vi "eventLogger.vi"() -> ()   [LabVIEW 2017]
panel:
  in  "stop":bool
  in  "enter":bool
  in  "Event text":string
  in  "Rat ID":string
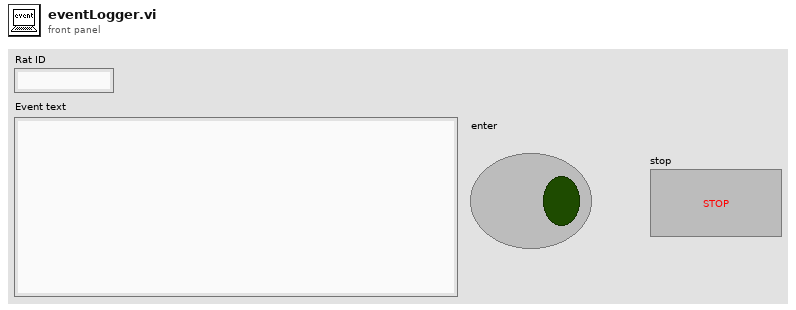
[diagram p1: front panel]
types:
  T1 = enum16{"open", "replace", "create", "open or create", "replace or create", "replace or create with confirmation"}
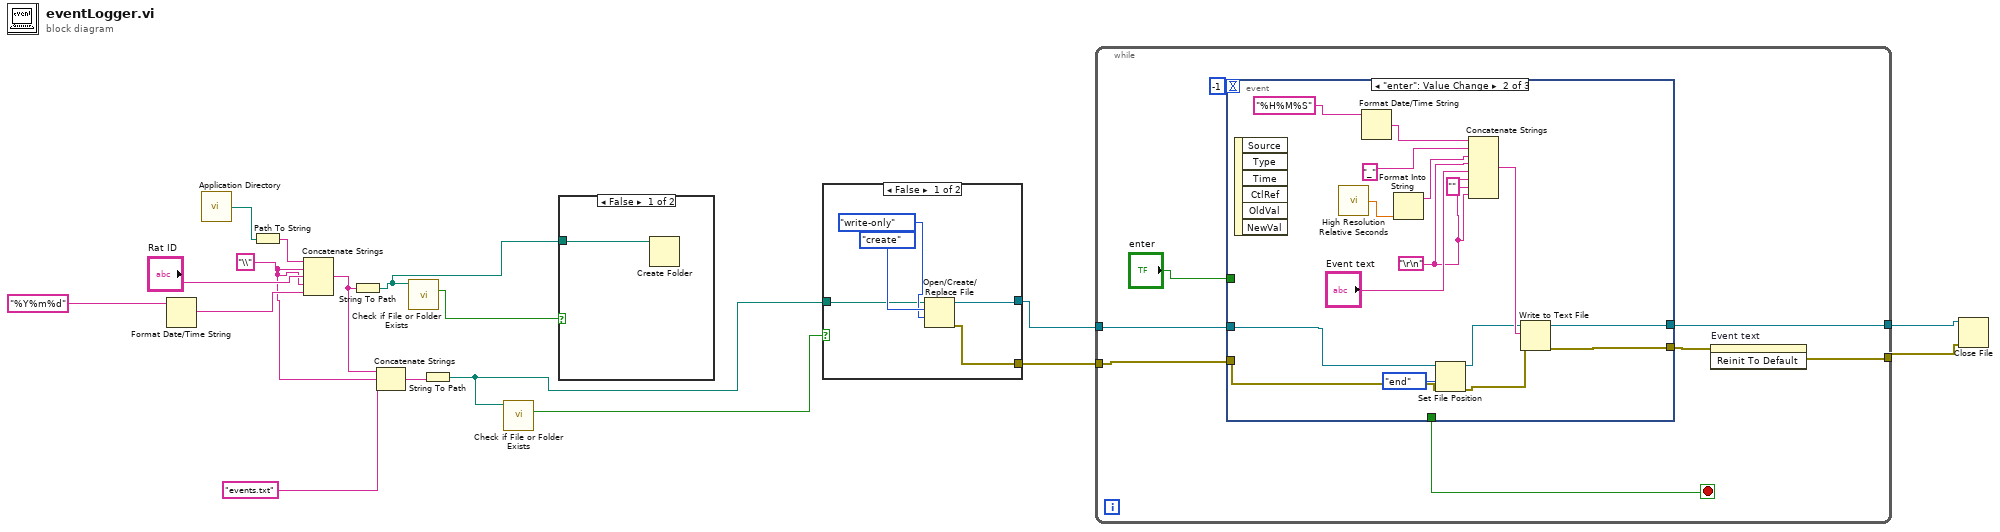
[diagram p0: block diagram]
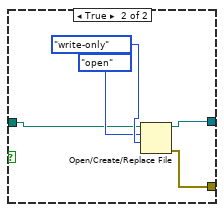
[diagram p2: hidden frame]
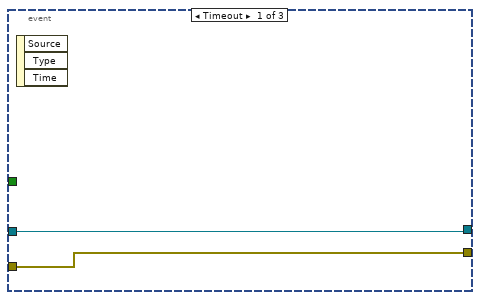
[diagram p4: hidden frame]
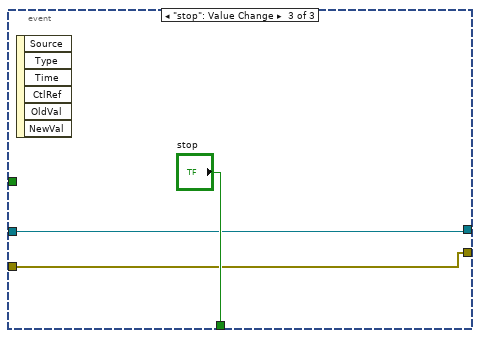
[diagram p5: hidden frame]
diagram:
  w12 = "\\" ("string")
  n1 = Format Date/Time String(time format string (%c)="%Y%m%d" ("time string")) -> (date/time string=w15:string)  [unwired: 2 in]
  n2 = call <vilib>:"Application Directory.vi"() -> ("Application Directory"=w14:path)
  n3 = Path To String(path=w14) -> (string=w17:string)
  n4 = Concatenate Strings(w17, w12, "Rat ID", w12, w15) -> (w11:string)
  n5 = String To Path(string=w11) -> (path=w7:path)
  n6 = Concatenate Strings(w11, w12, "events.txt" ("string")) -> (w9:string)
  n7 = call <vilib>:"Check if File or Folder Exists.vi"("path"=w7) -> ("file or folder exists?"=w8:bool)  [unwired: 8 in, 2 out]
  n8 = String To Path(string=w9) -> (path=w5:path)
  n9 = call <vilib>:"Check if File or Folder Exists.vi"("path"=w5) -> ("file or folder exists?"=w6:bool)  [unwired: 8 in, 2 out]
  n10 = case shown="False" w8 {
    tunnel: w7 -> [w18 _]
    frame False {
      n11 = Create Folder(path (use dialog)=w18) -> ()  [unwired: 2 in, 3 out]
    }
    frame True {
    }
  }
  n12 = case shown="False" w6 {
    tunnel: [w21 w25] -> w4
    tunnel: w5 -> [w20 w26]
    tunnel: [w19 w24] -> w3
    frame False {
      n13 = Open/Create/Replace File(file path (use dialog)=w20, operation (0:open)=T1."create", access (0:read/write)=enum16{"read/write", "read-only", "write-only"}."write-only") -> (refnum out=w21:refnum<file>, error out=w19:errorcluster)  [unwired: 3 in, 1 out]
    }
    frame True {
      n14 = Open/Create/Replace File(file path (use dialog)=w26, operation (0:open)=T1."open", access (0:read/write)=enum16{"read/write", "read-only", "write-only"}."write-only") -> (refnum out=w25:refnum<file>, error out=w24:errorcluster)  [unwired: 3 in, 1 out]
    }
  }
  n15 = while {
    tunnel: w4 -> [w30]
    tunnel: w3 -> [w36]
    tunnel: [w34] -> w2
    tunnel: [w29] -> w1
    stop <- w31 stop-if-true
    n16 = event shown="[1] \"enter\": Value Change" {
      selector: _ -> [_ _ _]
      dyn-events: _ -> [_ _ _]
      timeout: -1 -> [_ _ _]
      tunnel: w36 -> [w38 w49 w55]
      tunnel: [w38 w54 w55] -> w35
      tunnel: "enter" -> [_ _ _]
      tunnel: [_ _ "stop"] -> w31
      tunnel: w30 -> [w37 w46 w56]
      tunnel: [w37 w45 w56] -> w29
      event Timeout {
        n17 = event-data() -> ()  [unwired: 1 in, 3 out]
      }
      event "enter": Value Change {
        w39 = "\r\n"
        n18 = event-data() -> ()  [unwired: 1 in, 6 out]
        n19 = call <vilib>:"High Resolution Relative Seconds.vi"() -> ("relative seconds"=w53:dbl)
        n20 = Format Date/Time String(time format string (%c)="%H%M%S" ("time string")) -> (date/time string=w44:string)  [unwired: 2 in]
        n21 = Format Into String(w53) -> (resulting string=w52:string)  [unwired: 3 in, 1 out]
        n22 = Set File Position(refnum=w46, from (0:start)=enum16{"start", "end", "current"}."end", error in=w49) -> (refnum out=w48:refnum<file>, error out=w50:errorcluster)  [unwired: 1 in]
        n23 = Concatenate Strings(w44, "_" ("string"), w52, w39, "Event text", w39, "" ("string"), w39) -> (w51:string)
        n24 = Write to Text File(file (use dialog)=w48, text=w51, error in=w50) -> (refnum out=w45:refnum<file>, error out=w54:errorcluster)  [unwired: 1 in, 1 out]
      }
      event "stop": Value Change {
        n25 = event-data() -> ()  [unwired: 1 in, 6 out]
      }
    }
    n26 = invoke on="Event text" class="Str" method="Reinit To Default"(error in=w35) -> (error out=w34:errorcluster)  [unwired: 2 in, 2 out]
  }
  n27 = Close File(refnum=w1, error in=w2) -> ()  [unwired: 2 out]
